vi "DesiredStats2UniqueStats.vi"(11 "StatCluster In":string[][](array[string])) -> (3 "StatCluster Out":string[][](array[string]))   [LabVIEW 2013]
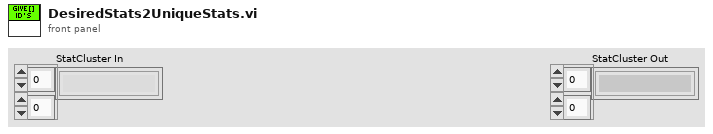
[diagram p1: front panel]
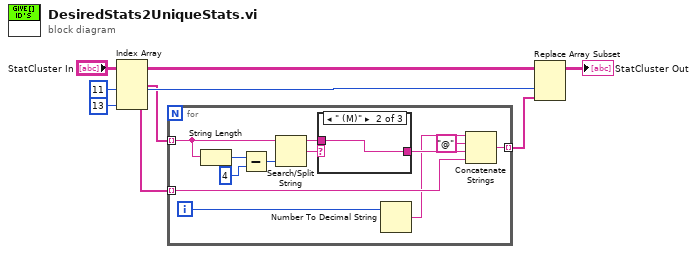
[diagram p0: block diagram]
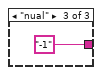
[diagram p3: hidden frame]
diagram:
  w6 = 11 ("disabled index (col)")
  n1 = Index Array(array="StatCluster In", index (col) #1=w6, index (col) #2=13 ("index (col)")) -> (element #1=w5:string[], element #2=w3:string[])  [unwired: 2 in]
  n2 = for {
    tunnel: w5 -> [w13] mode=indexing
    tunnel: w3 -> [w12] mode=indexing
    tunnel: [w8] -> w2 mode=indexing
    i -> [w9]
    n3 = String Length(string=w13) -> (length=w14:i32)
    n4 = Subtract(x=w14, y=4) -> (x-y=w17:i32)
    n5 = Search/Split String(string=w13, offset (0)=w17) -> (substring before match=w18:string, match + rest of string=w16:string)  [unwired: 1 in, 1 out]
    n6 = case shown="\" (M)\"" w16 {
      selector: w16 -> [w20 _ _]
      tunnel: [w20 w21 "-1"] -> w19
      tunnel: w18 -> [_ w21 _]
      frame Default {
      }
      frame " (M)" {
      }
      frame "nual" {
      }
    }
    n7 = Number To Decimal String(number=w9) -> (decimal integer string=w10:string)  [unwired: 1 in]
    n8 = Concatenate Strings(w10, "@" ("string"), w19, w12) -> (w8:string)
  }
  n9 = Replace Array Subset(array="StatCluster In", new element=w2, index (col)=w6) -> (→"StatCluster Out":string[][])  [unwired: 1 in]
